vi "FTW-Supervisor-Core-SerializeEvent.vi"(0 "Event Type":string, 5 "Event Data":string, 7 "Source":string, 11 "Error to Log":errorcluster) -> (4 "Serialized Event":string)   [LabVIEW 2015]
panel:
  # "Inputs"
  # "Outputs"
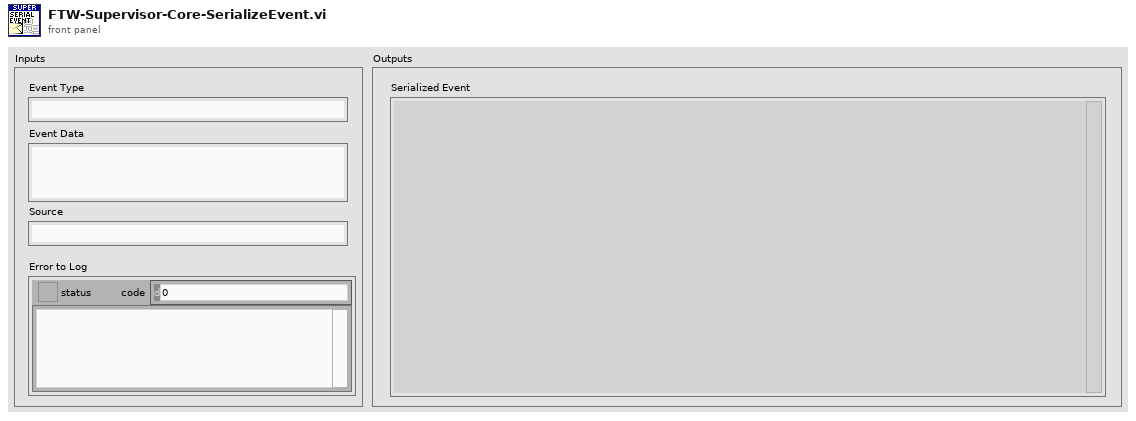
[diagram p1: front panel]
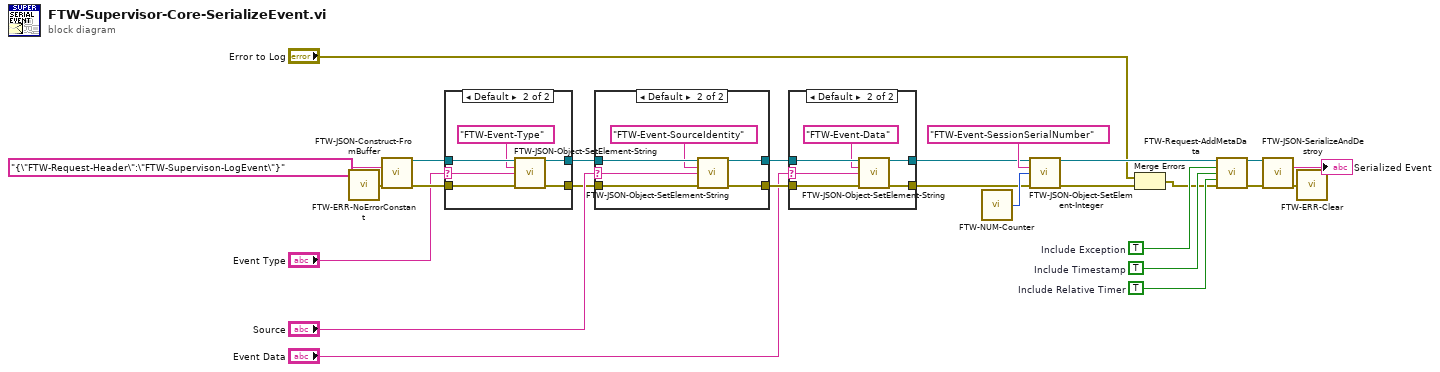
[diagram p0: block diagram]
diagram:
  w24 = TRUE  # Include Relative Timer
  w25 = TRUE  # Include Timestamp
  w26 = TRUE  # Include Exception
  n1 = call "FTW-ERR-NoErrorConstant.vi"() -> ("no error"=w18:errorcluster)
  n2 = call "FTW-JSON-Construct-FromBuffer.vi"("JSON String (UTF-8)"="{\"FTW-Request-Header\":\"FTW-Supervison-LogEvent\"}", "error in"=w18) -> ("JSON Object"=w5:refnum<data-value>, "error out"=w4:errorcluster)  [unwired: 12 in]
  n3 = case shown="Default" "Event Type" {
    selector: "Event Type" -> [_ w29]
    tunnel: w5 -> [w28 w34]
    tunnel: [w28 w33] -> w3
    tunnel: w4 -> [w27 w32]
    tunnel: [w27 w31] -> w2
    frame "" {
    }
    frame Default {
      n4 = call "FTW-JSON-Object-SetElement-String.vi"("JSON Object"=w34, "Key"="FTW-Event-Type", "Value"=w29, "error in"=w32) -> ("JSON Object out"=w33:refnum<data-value>, "error out"=w31:errorcluster)  [unwired: 10 in]
    }
  }
  n5 = case shown="Default" "Source" {
    selector: "Source" -> [_ w37]
    tunnel: w3 -> [w36 w42]
    tunnel: w2 -> [w35 w41]
    tunnel: [w36 w39] -> w11
    tunnel: [w35 w38] -> w9
    frame "" {
    }
    frame Default {
      n6 = call "FTW-JSON-Object-SetElement-String.vi"("JSON Object"=w42, "Key"="FTW-Event-SourceIdentity", "Value"=w37, "error in"=w41) -> ("JSON Object out"=w39:refnum<data-value>, "error out"=w38:errorcluster)  [unwired: 10 in]
    }
  }
  n7 = case shown="Default" "Event Data" {
    selector: "Event Data" -> [_ w45]
    tunnel: w11 -> [w44 w50]
    tunnel: [w44 w49] -> w10
    tunnel: w9 -> [w43 w48]
    tunnel: [w43 w47] -> w8
    frame "" {
    }
    frame Default {
      n8 = call "FTW-JSON-Object-SetElement-String.vi"("JSON Object"=w50, "Key"="FTW-Event-Data", "Value"=w45, "error in"=w48) -> ("JSON Object out"=w49:refnum<data-value>, "error out"=w47:errorcluster)  [unwired: 10 in]
    }
  }
  n9 = call "FTW-NUM-Counter.vi"() -> ("Counter"=w16:i32)  [unwired: 1 in]
  n10 = call "FTW-JSON-Object-SetElement-Integer.vi"("JSON Object"=w10, "Key"="FTW-Event-SessionSerialNumber", "Value"=w16, "error in"=w8) -> ("JSON Object out"=w15:refnum<data-value>, "error out"=w14:errorcluster)  [unwired: 10 in]
  n11 = Merge Errors("Error to Log", w14) -> (w13:errorcluster)
  n12 = call "FTW-Request-AddMetaData.vi"("Response"=w15, "Include Exception"=w26, "Include Timestamp"=w25, "Include Relative Timer"=w24, "error in"=w13) -> ("Response out"=w22:refnum<data-value>, "error out"=w20:errorcluster)  [unwired: 9 in]
  n13 = call "FTW-JSON-SerializeAndDestroy.vi"("JSON Object"=w22, "error in"=w20) -> ("JSON String (UTF-8)"=→"Serialized Event":string, "error out"=w19:errorcluster)  [unwired: 12 in]
  n14 = call "FTW-ERR-Clear.vi"("error to snuff"=w19) -> ()  [unwired: 1 out]
